vi "Run.vi"(8 "error in (no error)":errorcluster, 11 "Channel in":refnum<class "SPARC4_Channel.lvclass">) -> (0 "error out":errorcluster, 3 "Channel out":refnum<class "SPARC4_Channel.lvclass">)   [LabVIEW 2018, in "SPARC4_Channel.lvclass"]
doc: "Run the channel"
uses:
  SPARC4_Channel.lvclass
  C:/Users/Denis/Desktop/S4ACS/S4ACS/Channel/Channel.lvclass
  Channel/Channel.lvclass/Channel.ctl
  SPARC4_Channel.lvclass/SPARC4_Channel.ctl
  Sim_Ixon_Ultra/Sim_Ixon_Ultra.lvclass
  C:/Users/Denis/Desktop/S4ACS/S4ACS/Sim_CCD/Sim_CCD.lvclass
  State Machine/State Machine.lvclass
  Sim_CCD/Sim_CCD.lvclass
  RxTx/RxTx.lvclass
  Server/Server.lvclass
  Channel/Channel.lvclass
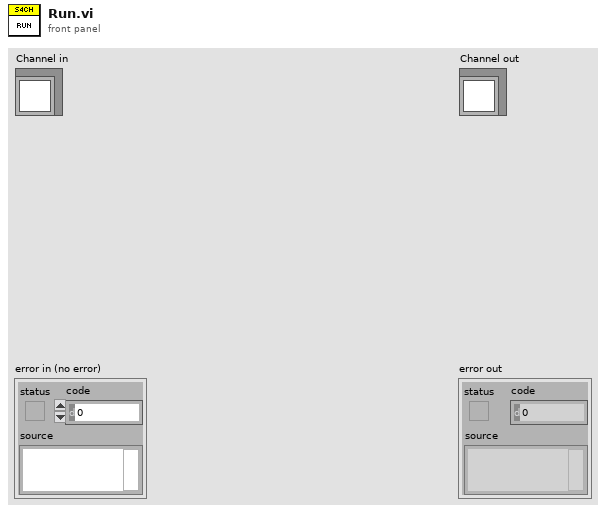
[diagram p1: front panel]
types:
  T1 = cluster{"State Machine.lvclass":refnum<class "State Machine.lvclass">, "RxTx.lvclass":refnum<class "RxTx.lvclass">, "Save_Header_RxTx.lvclass":refnum<class "RxTx.lvclass">, "Status SM.lvclass":refnum<class "State Machine.lvclass">, "Status RxTx.lvclass":refnum<class "RxTx.lvclass">, "servers array":refnum<class "Server.lvclass">[], "Events log file.lvclass":refnum<class "Log File.lvclass">, "Errors log file.lvclass":refnum<class "Log File.lvclass">, "Keywords log file.lvclass":refnum<class "Log File.lvclass">, "Sim_CCD.lvclass":refnum<class "Sim_CCD.lvclass">}
  T2 = cluster{"field 1":string, "field 2":string, "field 3":string}
  T3 = cluster{"PREAMP":u16, "READOUT_RATE":u16, "VERTICAL_SHIFT_SPEED":u16, "READ_MODE":u16, "VERTICAL_CLOCK_VOLTAGE":u16, "ACQUISITION_MODE":u16, "AD_CHANNEL":u16, "SHUTTER_TTL":u16, "SHUTTER_OPENING_TIME":u16, "SHUTTER_CLOSING_TIME":u16, "SHUTTER_MODE":u16, "TRIGGER_MODE":u16, "VBIN":u16, "INITIAL_LINE":u16, "INITIAL_COLUMN":u16, "FINAL_LINE":u16, "FINAL_COLUMN":u16, "HBIN":u16, "TEMP":i32, "COOLER_POWER_STATUS":u16}
  T4 = cluster{"EM_MODE":u16, "EM_GAIN":u16, "FRAME_TRANSFER":bool}
  T5 = typedef "LVDateTimeRec.ctl" = cluster{"fractional second":dbl, "second":i32, "minute":i32, "hour":i32, "day of month":i32, "month":i32, "year":i32, "day of week":i32, "day of year":i32, "DST":i32}
  T6 = cluster{"Time Acq Started":u32, "Image delay":u64, "Last update - CCD config":timestamp, "SYSTEMTIME":T5, "Readout time":dbl, "Time acq finished":u32, "effective exptime":dbl}
  T7 = cluster{"FRAMES_DONE":u16, "CCD_STATUS":string, "CURRENT_TEMPERATURE":i16, "TEMPERATURE_STATUS":string, "FRAME_EXPOSURE_TIME":sgl, "SERIAL_NUMBER":u16, "ACQUIRING":bool, "POWER":bool}
  T8 = cluster{"Stop Acquisition":bool, "Abort Acquisition":bool, "Pause acquisition":bool, "wait expose command":bool, "video mode":bool, "stop app":bool}
  T9 = cluster{"CYCLES_DONE":u16, "LAST_IMAGE_NAME":string, "USED_DISK_SPACE":u16, "IMAGE_INDEX":u32, "acquisition error":bool}
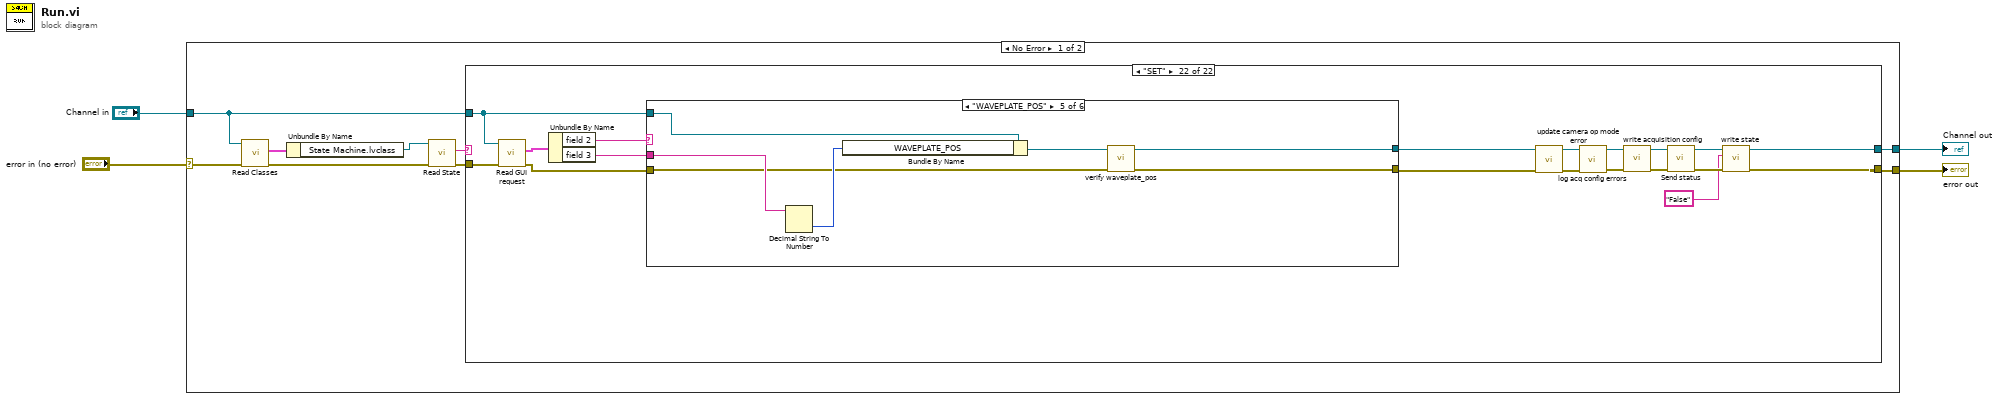
[diagram p0: block diagram]
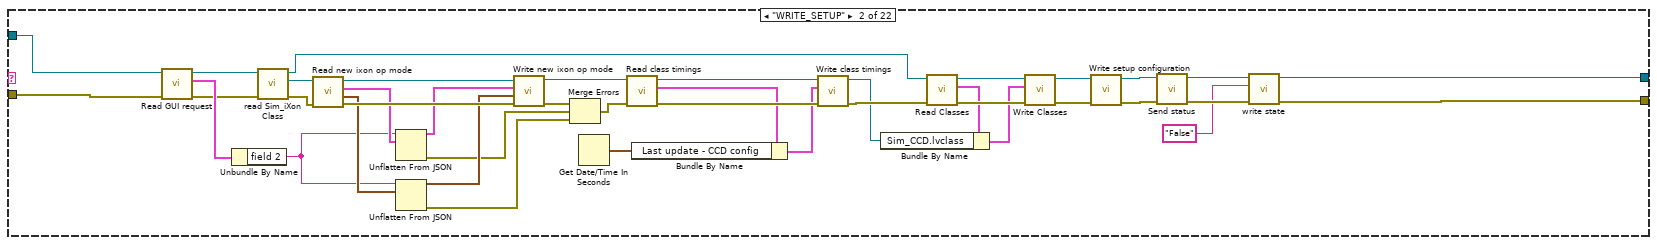
[diagram p3: hidden frame]
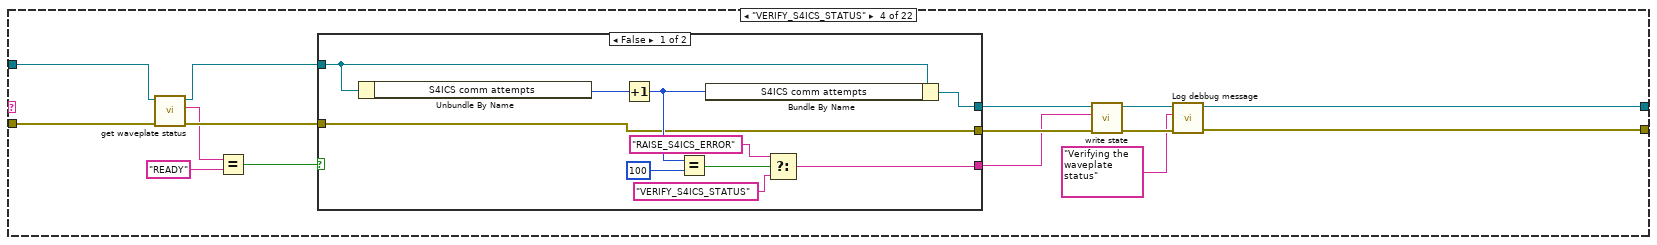
[diagram p5: hidden frame]
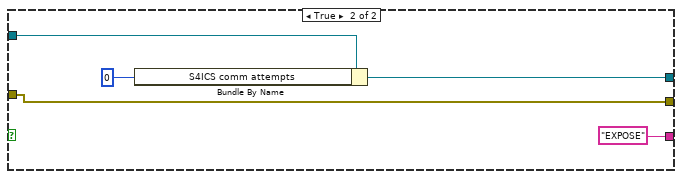
[diagram p6: hidden frame]
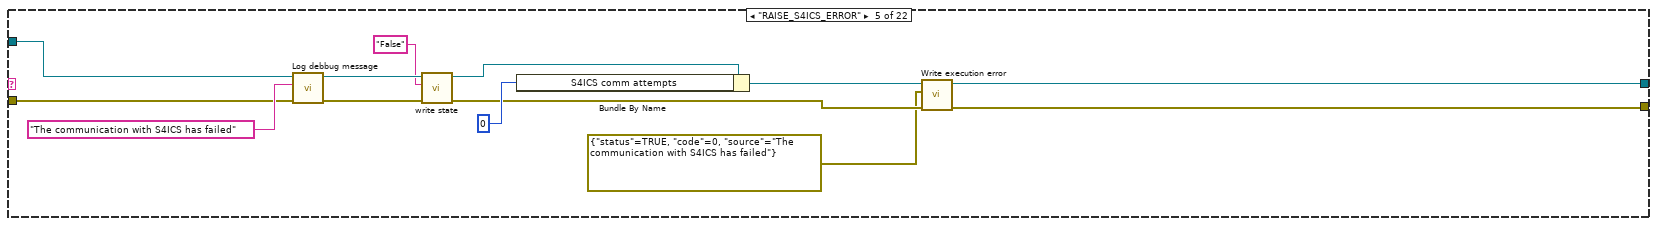
[diagram p7: hidden frame]
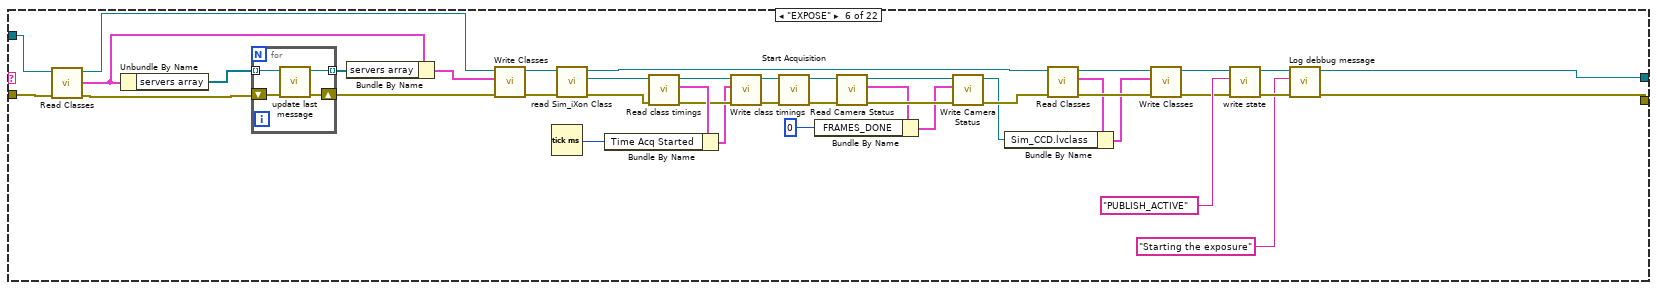
[diagram p8: hidden frame]
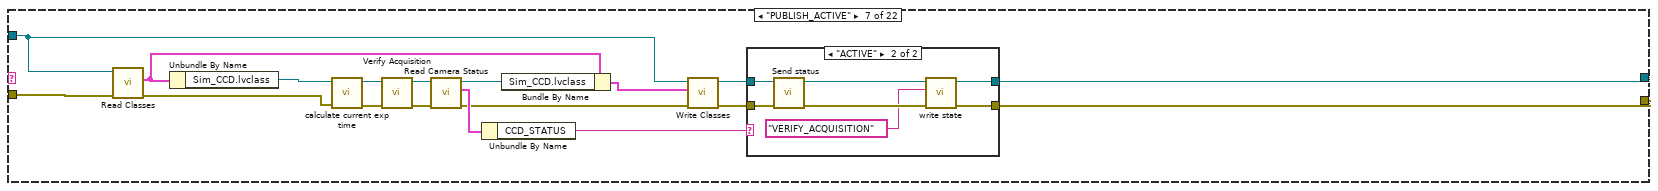
[diagram p9: hidden frame]
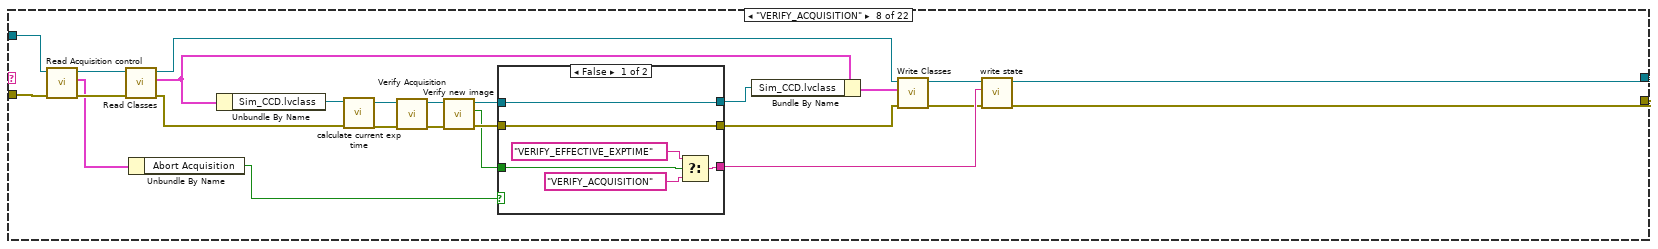
[diagram p11: hidden frame]
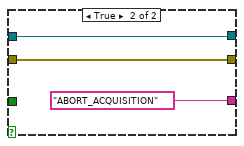
[diagram p12: hidden frame]
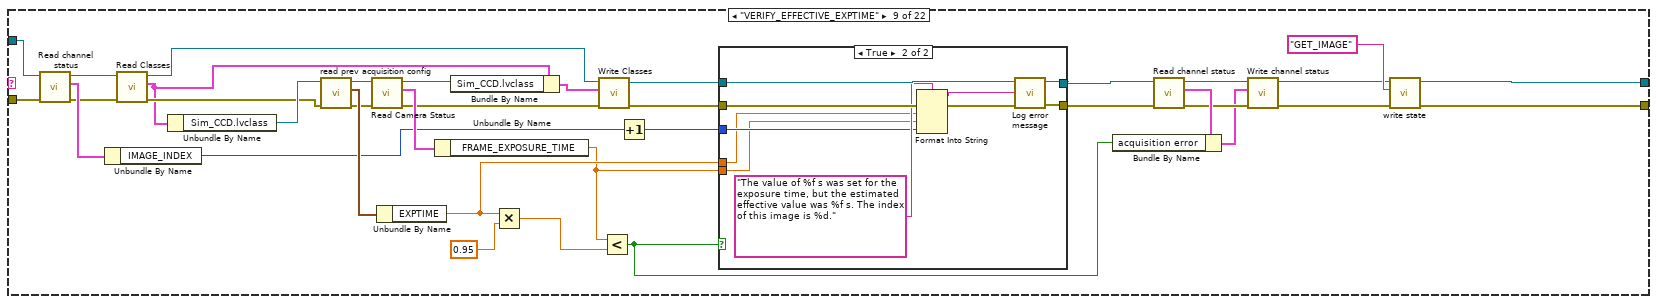
[diagram p13: hidden frame]
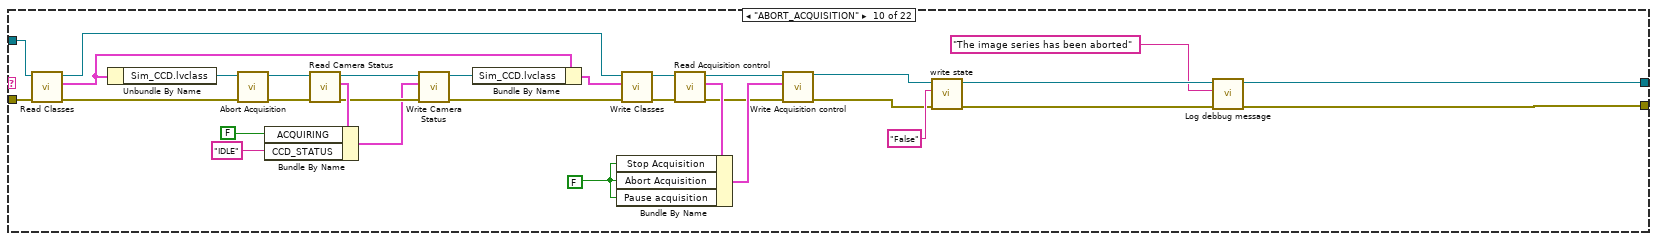
[diagram p15: hidden frame]
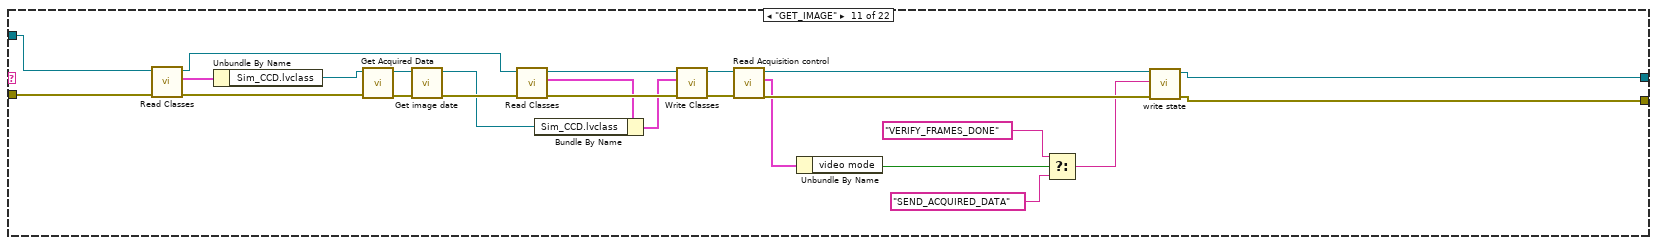
[diagram p16: hidden frame]
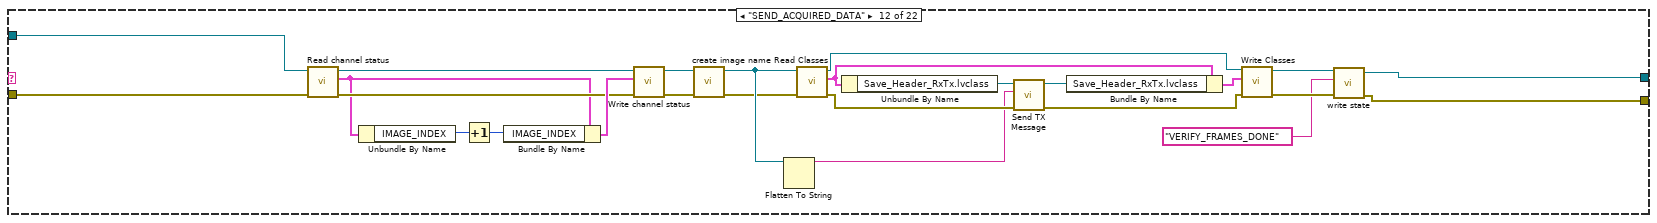
[diagram p17: hidden frame]
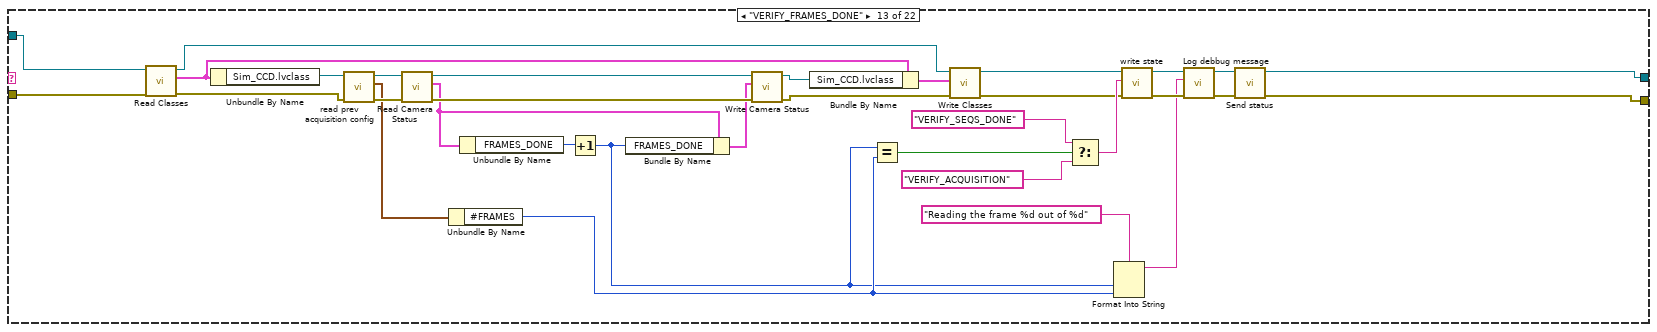
[diagram p18: hidden frame]
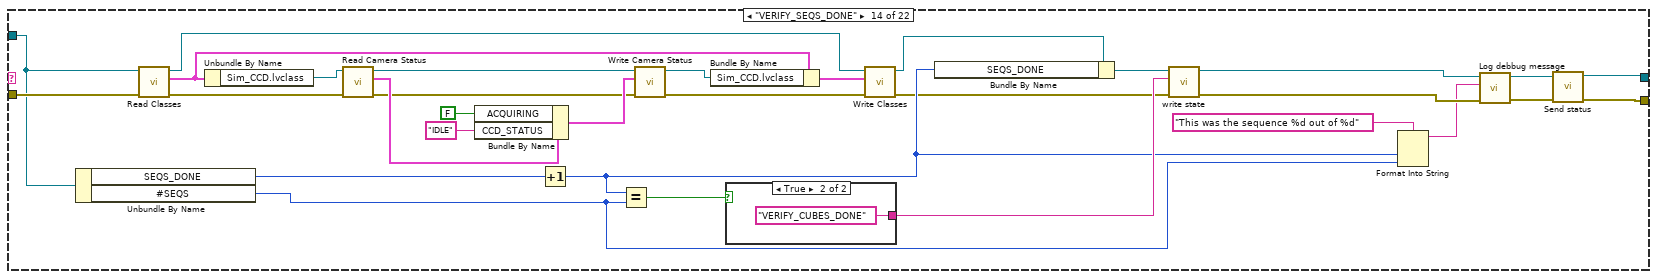
[diagram p19: hidden frame]
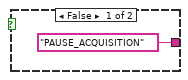
[diagram p20: hidden frame]
diagram:
  n1 = case shown="No Error" "error in (no error)" {
    selector: "error in (no error)" -> [w7 w611]
    tunnel: [w13 w611] -> w3
    tunnel: [w12 w610] -> w1
    tunnel: "Channel in" -> [w8 w610]
    frame No Error {
      n2 = call-dynamic "Read Classes.vi"("error in (no error)"=w7, "Channel in"=w8) -> ("error out"=w6:errorcluster, "Classes"=w9:T1)  [unwired: 7 in, 1 out]
      n3 = Unbundle By Name(w9) -> ("State Machine.lvclass"=w5:refnum<class "State Machine.lvclass">)
      n4 = call-dynamic "Read State.vi"("error in (no error)"=w6, "State Machine in"=w5) -> ("error out"=w11:errorcluster, "State"=w10:string)  [unwired: 7 in, 1 out]
      n5 = case shown="\"SET\"" w10 {
        tunnel: w11 -> [w14 w32 w56 w60 w98 w122 w156 w179 w220 w273 w307 w316 w360 w385 w410 w436 w440 w467 w492 w511 w517 w524]
        tunnel: [w14 w19 w56 w66 w89 w132 w163 w195 w242 w276 w298 w336 w359 w372 w422 w432 w446 w470 w498 w513 w517 w534] -> w13
        tunnel: [w15 w20 w57 w67 w90 w133 w164 w196 w243 w277 w297 w337 w358 w373 w421 w433 w445 w471 w497 w512 w518 w535] -> w12
        tunnel: w8 -> [w15 w34 w57 w62 w99 w121 w151 w177 w214 w272 w308 w317 w361 w381 w408 w437 w441 w468 w493 w510 w518 w523]
        frame "False", Default {
        }
        frame "WRITE_SETUP" {
          n6 = call "Read GUI request.vi"("error in (no error)"=w32, "Channel in"=w34) -> ("error out"=w33:errorcluster, "GUI request"=w39:T2, "Channel out"=w35:refnum<class "SPARC4_Channel.lvclass">)  [unwired: 7 in]
          n7 = Unbundle By Name(w39) -> ("field 2"=w38:string)
          n8 = call "read Sim_iXon Class.vi"("error in (no error)"=w33, "SPARC4_Channel in"=w35) -> ("error out"=w36:errorcluster, "Sim_Ixon_Ultra.lvclass"=w37:refnum<class "Sim_Ixon_Ultra.lvclass">, "SPARC4_Channel out"=w25:refnum<class "SPARC4_Channel.lvclass">)  [unwired: 7 in]
          n9 = call-dynamic "Read new ixon op mode.vi"("error in (no error)"=w36, "Sim_Ixon_Ultra in"=w37) -> ("error out"=w54:errorcluster, "new operation mode"=w53:T3, "new ixon op mode"=w45:T4, "Sim_Ixon_Ultra out"=w55:refnum<class "Sim_Ixon_Ultra.lvclass">)  [unwired: 6 in]
          n10 = Unflatten From JSON(JSON string=w38, type and defaults=w45) -> (value=w44:T4, error out=w41:errorcluster)  [unwired: 5 in]
          n11 = Unflatten From JSON(JSON string=w38, type and defaults=w53) -> (value=w52:T3, error out=w40:errorcluster)  [unwired: 5 in]
          n12 = call-dynamic "Write new ixon op mode.vi"("error in (no error)"=w54, "new operation mode"=w52, "new ixon op mode"=w44, "Sim_Ixon_Ultra in"=w55) -> ("error out"=w43:errorcluster, "Sim_Ixon_Ultra out"=w51:refnum<class "Sim_Ixon_Ultra.lvclass">)  [unwired: 6 in]
          n13 = Merge Errors(w43, w41, w40) -> (w42:errorcluster)
          n14 = Get Date/Time In Seconds() -> (seconds since 1Jan1904=w46:timestamp)
          n15 = call "Read class timings.vi"("error in (no error)"=w42, "Simulated Camera in"=w51) -> ("error out"=w49:errorcluster, "class timings"=w48:T6, "Simulated Camera out"=w50:refnum<class "Sim_Ixon_Ultra.lvclass">)  [unwired: 7 in]
          n16 = Bundle By Name(cluster=w48, "Last update - CCD config"=w46) -> (w47:T6)
          n17 = call "Write class timings.vi"("error in (no error)"=w49, "class timings"=w47, "Simulated Camera in"=w50) -> ("error out"=w29:errorcluster, "Simulated Camera out"=w27:refnum<class "Sim_Ixon_Ultra.lvclass">)  [unwired: 7 in]
          n18 = call-dynamic "Read Classes.vi"("error in (no error)"=w29, "Channel in"=w25) -> ("error out"=w30:errorcluster, "Classes"=w28:T1, "Channel out"=w31:refnum<class "SPARC4_Channel.lvclass">)  [unwired: 7 in]
          n19 = Bundle By Name(cluster=w28, "Sim_CCD.lvclass"=w27) -> (w26:T1)
          n20 = call-dynamic "Write Classes.vi"("error in (no error)"=w30, "Classes"=w26, "Channel in"=w31) -> ("error out"=w21:errorcluster, "Channel out"=w23:refnum<class "SPARC4_Channel.lvclass">)  [unwired: 7 in]
          n21 = call "Write setup configuration.vi"("error in (no error)"=w21, "Channel in"=w23) -> ("error out"=w22:errorcluster, "Channel out"=w24:refnum<class "SPARC4_Channel.lvclass">)  [unwired: 8 in]
          n22 = call-dynamic "Send status.vi"("error in (no error)"=w22, "Channel in"=w24) -> ("error out"=w17:errorcluster, "Channel out"=w18:refnum<class "SPARC4_Channel.lvclass">)  [unwired: 8 in]
          n23 = call "write state.vi"("error in (no error)"=w17, "state"="False", "Channel in"=w18) -> ("error out"=w19:errorcluster, "Channel out"=w20:refnum<class "SPARC4_Channel.lvclass">)  [unwired: 7 in]
        }
        frame "---------------------------------" {
        }
        frame "VERIFY_S4ICS_STATUS" {
          n24 = call "get waveplate status.vi"("error in (no error)"=w60, "Channel in"=w62) -> ("error out"=w59:errorcluster, "wp condition"=w58:string, "Channel out"=w61:refnum<class "SPARC4_Channel.lvclass">)  [unwired: 7 in]
          n25 = Equal?(x=w58, y="READY") -> (x = y?=w71:bool)
          n26 = case shown="False" w71 {
            tunnel: w61 -> [w82 w87]
            tunnel: w59 -> [w75 w86]
            tunnel: [w74 w85] -> w70
            tunnel: [w75 w86] -> w69
            tunnel: [w73 "EXPOSE" ("y")] -> w68
            frame False {
              n27 = Unbundle By Name(w82) -> ("S4ICS comm attempts"=w81:u8)
              n28 = Increment(x=w81) -> (x+1=w80:u8)
              n29 = Equal?(x=w80, y=100) -> (x = y?=w78:bool)
              n30 = Bundle By Name(cluster=w82, "S4ICS comm attempts"=w80) -> (w74:refnum<class "SPARC4_Channel.lvclass">)
              n31 = Select(t="RAISE_S4ICS_ERROR" ("y"), s=w78, f="VERIFY_S4ICS_STATUS" ("y")) -> (s? t:f=w73:string)
            }
            frame True {
              n32 = Bundle By Name(cluster=w87, "S4ICS comm attempts"=u8 0) -> (w85:refnum<class "SPARC4_Channel.lvclass">)
            }
          }
          n33 = call "write state.vi"("error in (no error)"=w69, "state"=w68, "Channel in"=w70) -> ("error out"=w65:errorcluster, "Channel out"=w64:refnum<class "SPARC4_Channel.lvclass">)  [unwired: 7 in]
          n34 = call "Log debbug message.vi"("error in (no error)"=w65, "String"="Verifying the waveplate status" ("y"), "Channel in"=w64) -> ("error out"=w66:errorcluster, "Channel out"=w67:refnum<class "SPARC4_Channel.lvclass">)  [unwired: 7 in]
        }
        frame "RAISE_S4ICS_ERROR" {
          n35 = call "Log debbug message.vi"("error in (no error)"=w98, "String"="The communication with S4ICS has failed", "Channel in"=w99) -> ("error out"=w95:errorcluster, "Channel out"=w96:refnum<class "SPARC4_Channel.lvclass">)  [unwired: 7 in]
          n36 = call "write state.vi"("error in (no error)"=w95, "state"="False", "Channel in"=w96) -> ("error out"=w91:errorcluster, "Channel out"=w94:refnum<class "SPARC4_Channel.lvclass">)  [unwired: 7 in]
          n37 = Bundle By Name(cluster=w94, "S4ICS comm attempts"=u8 0) -> (w92:refnum<class "SPARC4_Channel.lvclass">)
          n38 = call-dynamic "Write execution error.vi"("error in (no error)"=w91, "execution error"=errorcluster {"status"=TRUE, "code"=0, "source"="The communication with S4ICS has failed"} ("error constant"), "Channel in"=w92) -> ("error out"=w89:errorcluster, "Channel out"=w90:refnum<class "SPARC4_Channel.lvclass">)  [unwired: 7 in]
        }
        frame "EXPOSE" {
          n39 = call-dynamic "Read Classes.vi"("error in (no error)"=w122, "Channel in"=w121) -> ("error out"=w118:errorcluster, "Classes"=w115:T1, "Channel out"=w119:refnum<class "SPARC4_Channel.lvclass">)  [unwired: 7 in]
          n40 = Unbundle By Name(w115) -> ("servers array"=w120:refnum<class "Server.lvclass">[])
          n41 = for {
            tunnel: w120 -> [w143] mode=indexing
            shift-right: [w146] -> w117
            shift-left: w118 -> [w144]
            tunnel: [w145] -> w114 mode=indexing
            n42 = call "update last message.vi"("error in (no error)"=w144, "Server in"=w143) -> ("error out"=w146:errorcluster, "Server out"=w145:refnum<class "Server.lvclass">)  [unwired: 8 in]
          }
          n43 = Bundle By Name(cluster=w115, "servers array"=w114) -> (w116:T1)
          n44 = call-dynamic "Write Classes.vi"("error in (no error)"=w117, "Classes"=w116, "Channel in"=w119) -> ("error out"=w111:errorcluster, "Channel out"=w112:refnum<class "SPARC4_Channel.lvclass">)  [unwired: 7 in]
          n45 = Tick Count (ms)() -> (millisecond timer value=w123:u32)
          n46 = call "read Sim_iXon Class.vi"("error in (no error)"=w111, "SPARC4_Channel in"=w112) -> ("error out"=w110:errorcluster, "Sim_Ixon_Ultra.lvclass"=w113:refnum<class "Sim_Ixon_Ultra.lvclass">, "SPARC4_Channel out"=w104:refnum<class "SPARC4_Channel.lvclass">)  [unwired: 7 in]
          n47 = call "Read class timings.vi"("error in (no error)"=w110, "Simulated Camera in"=w113) -> ("error out"=w126:errorcluster, "class timings"=w127:T6, "Simulated Camera out"=w125:refnum<class "Sim_Ixon_Ultra.lvclass">)  [unwired: 7 in]
          n48 = Bundle By Name(cluster=w127, "Time Acq Started"=w123) -> (w124:T6)
          n49 = call "Write class timings.vi"("error in (no error)"=w126, "class timings"=w124, "Simulated Camera in"=w125) -> ("error out"=w129:errorcluster, "Simulated Camera out"=w128:refnum<class "Sim_Ixon_Ultra.lvclass">)  [unwired: 7 in]
          n50 = call-dynamic "Start Acquisition.vi"("error in (no error)"=w129, "CCDCamera in"=w128) -> ("error out"=w135:errorcluster, "CCDCamera out"=w136:refnum<class "Sim_Ixon_Ultra.lvclass">)  [unwired: 8 in]
          n51 = call "Read Camera Status.vi"("error in (no error)"=w135, "CCDCamera in"=w136) -> ("error out"=w142:errorcluster, "camera status"=w140:T7, "CCDCamera out"=w141:refnum<class "Sim_Ixon_Ultra.lvclass">)  [unwired: 7 in]
          n52 = Bundle By Name(cluster=w140, "FRAMES_DONE"=u16 0) -> (w139:T7)
          n53 = call "Write Camera Status.vi"("error in (no error)"=w142, "camera status"=w139, "CCDCamera in"=w141) -> ("error out"=w109:errorcluster, "CCDCamera out"=w101:refnum<class "Sim_Ixon_Ultra.lvclass">)  [unwired: 7 in]
          n54 = call-dynamic "Read Classes.vi"("error in (no error)"=w109, "Channel in"=w104) -> ("error out"=w106:errorcluster, "Classes"=w103:T1, "Channel out"=w105:refnum<class "SPARC4_Channel.lvclass">)  [unwired: 7 in]
          n55 = Bundle By Name(cluster=w103, "Sim_CCD.lvclass"=w101) -> (w102:T1)
          n56 = call-dynamic "Write Classes.vi"("error in (no error)"=w106, "Classes"=w102, "Channel in"=w105) -> ("error out"=w108:errorcluster, "Channel out"=w107:refnum<class "SPARC4_Channel.lvclass">)  [unwired: 7 in]
          n57 = call "write state.vi"("error in (no error)"=w108, "state"="PUBLISH_ACTIVE", "Channel in"=w107) -> ("error out"=w131:errorcluster, "Channel out"=w134:refnum<class "SPARC4_Channel.lvclass">)  [unwired: 7 in]
          n58 = call "Log debbug message.vi"("error in (no error)"=w131, "String"="Starting the exposure", "Channel in"=w134) -> ("error out"=w132:errorcluster, "Channel out"=w133:refnum<class "SPARC4_Channel.lvclass">)  [unwired: 7 in]
        }
        frame "PUBLISH_ACTIVE" {
          n59 = call-dynamic "Read Classes.vi"("error in (no error)"=w156, "Channel in"=w151) -> ("error out"=w154:errorcluster, "Classes"=w149:T1)  [unwired: 7 in, 1 out]
          n60 = Unbundle By Name(w149) -> ("Sim_CCD.lvclass"=w155:refnum<class "Sim_CCD.lvclass">)
          n61 = call-dynamic "calculate current exp time.vi"("error in (no error)"=w154, "CCDCamera in"=w155) -> ("error out"=w157:errorcluster, "CCDCamera out"=w158:refnum<class "Sim_CCD.lvclass">)  [unwired: 8 in]
          n62 = call-dynamic "Verify Acquisition.vi"("error in (no error)"=w157, "CCDCamera in"=w158) -> ("error out"=w159:errorcluster, "CCDCamera out"=w160:refnum<class "Sim_CCD.lvclass">)  [unwired: 8 in]
          n63 = call "Read Camera Status.vi"("error in (no error)"=w159, "CCDCamera in"=w160) -> ("error out"=w150:errorcluster, "camera status"=w162:T7, "CCDCamera out"=w148:refnum<class "Sim_CCD.lvclass">)  [unwired: 7 in]
          n64 = Unbundle By Name(w162) -> ("CCD_STATUS"=w161:string)
          n65 = Bundle By Name(cluster=w149, "Sim_CCD.lvclass"=w148) -> (w147:T1)
          n66 = call-dynamic "Write Classes.vi"("error in (no error)"=w150, "Classes"=w147, "Channel in"=w151) -> ("error out"=w152:errorcluster, "Channel out"=w153:refnum<class "SPARC4_Channel.lvclass">)  [unwired: 7 in]
          n67 = case shown="\"ACTIVE\"" w161 {
            tunnel: w153 -> [w166 w169]
            tunnel: [w166 w173] -> w164
            tunnel: [w165 w172] -> w163
            tunnel: w152 -> [w165 w168]
            frame "False", Default {
            }
            frame "ACTIVE" {
              n68 = call-dynamic "Send status.vi"("error in (no error)"=w168, "Channel in"=w169) -> ("error out"=w171:errorcluster, "Channel out"=w170:refnum<class "SPARC4_Channel.lvclass">)  [unwired: 8 in]
              n69 = call "write state.vi"("error in (no error)"=w171, "state"="VERIFY_ACQUISITION", "Channel in"=w170) -> ("error out"=w172:errorcluster, "Channel out"=w173:refnum<class "SPARC4_Channel.lvclass">)  [unwired: 7 in]
            }
          }
        }
        frame "VERIFY_ACQUISITION" {
          n70 = call "Read Acquisition control.vi"("error in (no error)"=w179, "Channel in"=w177) -> ("error out"=w178:errorcluster, "Acquisition control"=w175:T8, "Channel out"=w176:refnum<class "SPARC4_Channel.lvclass">)  [unwired: 7 in]
          n71 = call-dynamic "Read Classes.vi"("error in (no error)"=w178, "Channel in"=w176) -> ("error out"=w185:errorcluster, "Classes"=w182:T1, "Channel out"=w184:refnum<class "SPARC4_Channel.lvclass">)  [unwired: 7 in]
          n72 = Unbundle By Name(w175) -> ("Abort Acquisition"=w174:bool)
          n73 = Unbundle By Name(w182) -> ("Sim_CCD.lvclass"=w183:refnum<class "Sim_CCD.lvclass">)
          n74 = call-dynamic "calculate current exp time.vi"("error in (no error)"=w185, "CCDCamera in"=w183) -> ("error out"=w191:errorcluster, "CCDCamera out"=w192:refnum<class "Sim_CCD.lvclass">)  [unwired: 8 in]
          n75 = call-dynamic "Verify Acquisition.vi"("error in (no error)"=w191, "CCDCamera in"=w192) -> ("error out"=w198:errorcluster, "CCDCamera out"=w197:refnum<class "Sim_CCD.lvclass">)  [unwired: 8 in]
          n76 = call-dynamic "Verify new image.vi"("error in (no error)"=w198, "CCDCamera in"=w197) -> ("error out"=w193:errorcluster, "New Images ?"=w189:bool, "CCDCamera out"=w194:refnum<class "Sim_CCD.lvclass">)  [unwired: 7 in]
          n77 = case shown="False" w174 {
            tunnel: w194 -> [w204 w207]
            tunnel: w193 -> [w203 w206]
            tunnel: [w204 w207] -> w180
            tunnel: [w203 w206] -> w186
            tunnel: [w200 "ABORT_ACQUISITION"] -> w190
            tunnel: w189 -> [w199 _]
            frame False {
              n78 = Select(t="VERIFY_EFFECTIVE_EXPTIME", s=w199, f="VERIFY_ACQUISITION") -> (s? t:f=w200:string)
            }
            frame True {
            }
          }
          n79 = Bundle By Name(cluster=w182, "Sim_CCD.lvclass"=w180) -> (w181:T1)
          n80 = call-dynamic "Write Classes.vi"("error in (no error)"=w186, "Classes"=w181, "Channel in"=w184) -> ("error out"=w188:errorcluster, "Channel out"=w187:refnum<class "SPARC4_Channel.lvclass">)  [unwired: 7 in]
          n81 = call "write state.vi"("error in (no error)"=w188, "state"=w190, "Channel in"=w187) -> ("error out"=w195:errorcluster, "Channel out"=w196:refnum<class "SPARC4_Channel.lvclass">)  [unwired: 7 in]
        }
        frame "VERIFY_EFFECTIVE_EXPTIME" {
          n82 = call-dynamic "Read channel status.vi"("error in (no error)"=w220, "Channel in"=w214) -> ("error out"=w219:errorcluster, "channel status"=w222:T9, "Channel out"=w218:refnum<class "SPARC4_Channel.lvclass">)  [unwired: 7 in]
          n83 = Unbundle By Name(w222) -> ("IMAGE_INDEX"=w221:u32)
          n84 = call-dynamic "Read Classes.vi"("error in (no error)"=w219, "Channel in"=w218) -> ("error out"=w216:errorcluster, "Classes"=w210:T1, "Channel out"=w213:refnum<class "SPARC4_Channel.lvclass">)  [unwired: 7 in]
          n85 = Unbundle By Name(w210) -> ("Sim_CCD.lvclass"=w217:refnum<class "Sim_CCD.lvclass">)
          n86 = call "read prev acquisition config.vi"("error in (no error)"=w216, "Simulated_CCD_Camera in"=w217) -> ("error out"=w236:errorcluster, "Prev SET parameters"=w238:cluster{"EXPTIME":dbl, "#FRAMES":u32}, "Simulated_CCD_Camera out"=w237:refnum<class "Sim_CCD.lvclass">)  [unwired: 7 in]
          n87 = call "Read Camera Status.vi"("error in (no error)"=w236, "CCDCamera in"=w237) -> ("error out"=w211:errorcluster, "camera status"=w235:T7, "CCDCamera out"=w208:refnum<class "Sim_CCD.lvclass">)  [unwired: 7 in]
          n88 = Unbundle By Name(w238) -> ("EXPTIME"=w233:dbl)
          n89 = Unbundle By Name(w235) -> ("FRAME_EXPOSURE_TIME"=w232:sgl)
          n90 = Bundle By Name(cluster=w210, "Sim_CCD.lvclass"=w208) -> (w209:T1)
          n91 = Multiply(x=w233, y=0.95) -> (x*y=w239:dbl)
          n92 = call-dynamic "Write Classes.vi"("error in (no error)"=w211, "Classes"=w209, "Channel in"=w213) -> ("error out"=w215:errorcluster, "Channel out"=w212:refnum<class "SPARC4_Channel.lvclass">)  [unwired: 7 in]
          n93 = Less?(x=w232, y=w239) -> (x < y?=w230:bool)
          n94 = Increment(x=w221) -> (x+1=w234:u32)
          n95 = case shown="True" w230 {
            tunnel: w212 -> [w245 w255]
            tunnel: [w245 w254] -> w229
            tunnel: [w244 w253] -> w228
            tunnel: w215 -> [w244 w252]
            tunnel: w234 -> [_ w248]
            tunnel: w233 -> [_ w247]
            tunnel: w232 -> [_ w246]
            frame False {
            }
            frame True {
              n96 = Format Into String(format string="The value of %f s was set for the exposure time, but the estimated effective value was %f s. The index of this image is %d.", error in=w252, w247, w246, w248) -> (resulting string=w249:string, error out=w251:errorcluster)  [unwired: 1 in]
              n97 = call "Log error message.vi"("error in (no error)"=w251, "String"=w249, "Channel in"=w255) -> ("error out"=w253:errorcluster, "Channel out"=w254:refnum<class "SPARC4_Channel.lvclass">)  [unwired: 7 in]
            }
          }
          n98 = call-dynamic "Read channel status.vi"("error in (no error)"=w228, "Channel in"=w229) -> ("error out"=w224:errorcluster, "channel status"=w231:T9, "Channel out"=w225:refnum<class "SPARC4_Channel.lvclass">)  [unwired: 7 in]
          n99 = Bundle By Name(cluster=w231, "acquisition error"=w230) -> (w223:T9)
          n100 = call-dynamic "Write channel status.vi"("error in (no error)"=w224, "channel status"=w223, "Channel in"=w225) -> ("error out"=w227:errorcluster, "Channel out"=w226:refnum<class "SPARC4_Channel.lvclass">)  [unwired: 7 in]
          n101 = call "write state.vi"("error in (no error)"=w227, "state"="GET_IMAGE", "Channel in"=w226) -> ("error out"=w242:errorcluster, "Channel out"=w243:refnum<class "SPARC4_Channel.lvclass">)  [unwired: 7 in]
        }
        frame "ABORT_ACQUISITION" {
          w256 = FALSE ("Acquiring")
          n102 = call-dynamic "Read Classes.vi"("error in (no error)"=w273, "Channel in"=w272) -> ("error out"=w270:errorcluster, "Classes"=w266:T1, "Channel out"=w265:refnum<class "SPARC4_Channel.lvclass">)  [unwired: 7 in]
          n103 = Unbundle By Name(w266) -> ("Sim_CCD.lvclass"=w271:refnum<class "Sim_CCD.lvclass">)
          n104 = call-dynamic "Abort Acquisition.vi"("error in (no error)"=w270, "CCDCamera in"=w271) -> ("error out"=w284:errorcluster, "CCDCamera out"=w285:refnum<class "Sim_CCD.lvclass">)  [unwired: 8 in]
          n105 = call "Read Camera Status.vi"("error in (no error)"=w284, "CCDCamera in"=w285) -> ("error out"=w282:errorcluster, "camera status"=w287:T7, "CCDCamera out"=w283:refnum<class "Sim_CCD.lvclass">)  [unwired: 7 in]
          n106 = Bundle By Name(cluster=w287, "ACQUIRING"=FALSE ("Acquiring"), "CCD_STATUS"="IDLE" ("STATUS")) -> (w281:T7)
          n107 = call "Write Camera Status.vi"("error in (no error)"=w282, "camera status"=w281, "CCDCamera in"=w283) -> ("error out"=w268:errorcluster, "CCDCamera out"=w269:refnum<class "Sim_CCD.lvclass">)  [unwired: 7 in]
          n108 = Bundle By Name(cluster=w266, "Sim_CCD.lvclass"=w269) -> (w267:T1)
          n109 = call-dynamic "Write Classes.vi"("error in (no error)"=w268, "Classes"=w267, "Channel in"=w265) -> ("error out"=w263:errorcluster, "Channel out"=w264:refnum<class "SPARC4_Channel.lvclass">)  [unwired: 7 in]
          n110 = call "Read Acquisition control.vi"("error in (no error)"=w263, "Channel in"=w264) -> ("error out"=w257:errorcluster, "Acquisition control"=w259:T8, "Channel out"=w262:refnum<class "SPARC4_Channel.lvclass">)  [unwired: 7 in]
          n111 = Bundle By Name(cluster=w259, "Stop Acquisition"=w256, "Abort Acquisition"=w256, "Pause acquisition"=w256) -> (w258:T8)
          n112 = call "Write Acquisition control.vi"("error in (no error)"=w257, "Acquisition control"=w258, "Channel in"=w262) -> ("error out"=w260:errorcluster, "Channel out"=w261:refnum<class "SPARC4_Channel.lvclass">)  [unwired: 7 in]
          n113 = call "write state.vi"("error in (no error)"=w260, "state"="False", "Channel in"=w261) -> ("error out"=w275:errorcluster, "Channel out"=w278:refnum<class "SPARC4_Channel.lvclass">)  [unwired: 7 in]
          n114 = call "Log debbug message.vi"("error in (no error)"=w275, "String"="The image series has been aborted", "Channel in"=w278) -> ("error out"=w276:errorcluster, "Channel out"=w277:refnum<class "SPARC4_Channel.lvclass">)  [unwired: 7 in]
        }
        frame "GET_IMAGE" {
          n115 = call-dynamic "Read Classes.vi"("error in (no error)"=w307, "Channel in"=w308) -> ("error out"=w305:errorcluster, "Classes"=w306:T1, "Channel out"=w303:refnum<class "SPARC4_Channel.lvclass">)  [unwired: 7 in]
          n116 = Unbundle By Name(w306) -> ("Sim_CCD.lvclass"=w304:refnum<class "Sim_CCD.lvclass">)
          n117 = call-dynamic "Get Acquired Data.vi"("error in (no error)"=w305, "CCDCamera in"=w304) -> ("error out"=w311:errorcluster, "CCDCamera out"=w312:refnum<class "Sim_CCD.lvclass">)  [unwired: 8 in]
          n118 = call-dynamic "Get image date.vi"("error in (no error)"=w311, "Simulated_CCD_Camera in"=w312) -> ("error out"=w310:errorcluster, "Simulated_CCD_Camera out"=w309:refnum<class "Sim_CCD.lvclass">)  [unwired: 8 in]
          n119 = call-dynamic "Read Classes.vi"("error in (no error)"=w310, "Channel in"=w303) -> ("error out"=w302:errorcluster, "Classes"=w301:T1, "Channel out"=w300:refnum<class "SPARC4_Channel.lvclass">)  [unwired: 7 in]
          n120 = Bundle By Name(cluster=w301, "Sim_CCD.lvclass"=w309) -> (w299:T1)
          n121 = call-dynamic "Write Classes.vi"("error in (no error)"=w302, "Classes"=w299, "Channel in"=w300) -> ("error out"=w295:errorcluster, "Channel out"=w296:refnum<class "SPARC4_Channel.lvclass">)  [unwired: 7 in]
          n122 = call "Read Acquisition control.vi"("error in (no error)"=w295, "Channel in"=w296) -> ("error out"=w293:errorcluster, "Acquisition control"=w292:T8, "Channel out"=w294:refnum<class "SPARC4_Channel.lvclass">)  [unwired: 7 in]
          n123 = Unbundle By Name(w292) -> ("video mode"=w291:bool)
          n124 = Select(t="VERIFY_FRAMES_DONE", s=w291, f="SEND_ACQUIRED_DATA") -> (s? t:f=w288:string)
          n125 = call "write state.vi"("error in (no error)"=w293, "state"=w288, "Channel in"=w294) -> ("error out"=w298:errorcluster, "Channel out"=w297:refnum<class "SPARC4_Channel.lvclass">)  [unwired: 7 in]
        }
        frame "SEND_ACQUIRED_DATA" {
          n126 = call-dynamic "Read channel status.vi"("error in (no error)"=w316, "Channel in"=w317) -> ("error out"=w323:errorcluster, "channel status"=w315:T9, "Channel out"=w322:refnum<class "SPARC4_Channel.lvclass">)  [unwired: 7 in]
          n127 = Unbundle By Name(w315) -> ("IMAGE_INDEX"=w314:u32)
          n128 = Increment(x=w314) -> (x+1=w313:u32)
          n129 = Bundle By Name(cluster=w315, "IMAGE_INDEX"=w313) -> (w324:T9)
          n130 = call-dynamic "Write channel status.vi"("error in (no error)"=w323, "channel status"=w324, "Channel in"=w322) -> ("error out"=w318:errorcluster, "Channel out"=w319:refnum<class "SPARC4_Channel.lvclass">)  [unwired: 7 in]
          n131 = call-dynamic "create image name.vi"("error in (no error)"=w318, "Channel in"=w319) -> ("error out"=w320:errorcluster, "Channel out"=w321:refnum<class "SPARC4_Channel.lvclass">)  [unwired: 8 in]
          n132 = Flatten To String(anything=w321) -> (data string=w326:string)  [unwired: 3 in, 2 out]
          n133 = call-dynamic "Read Classes.vi"("error in (no error)"=w320, "Channel in"=w321) -> ("error out"=w331:errorcluster, "Classes"=w330:T1, "Channel out"=w325:refnum<class "SPARC4_Channel.lvclass">)  [unwired: 7 in]
          n134 = Unbundle By Name(w330) -> ("Save_Header_RxTx.lvclass"=w332:refnum<class "RxTx.lvclass">)
          n135 = call "Send TX Message.vi"("error in (no error)"=w331, "message"=w326, "RxTx in"=w332) -> ("error out"=w327:errorcluster, "RxTx out"=w328:refnum<class "RxTx.lvclass">)  [unwired: 7 in]
          n136 = Bundle By Name(cluster=w330, "Save_Header_RxTx.lvclass"=w328) -> (w329:T1)
          n137 = call-dynamic "Write Classes.vi"("error in (no error)"=w327, "Classes"=w329, "Channel in"=w325) -> ("error out"=w335:errorcluster, "Channel out"=w334:refnum<class "SPARC4_Channel.lvclass">)  [unwired: 7 in]
          n138 = call "write state.vi"("error in (no error)"=w335, "state"="VERIFY_FRAMES_DONE", "Channel in"=w334) -> ("error out"=w336:errorcluster, "Channel out"=w337:refnum<class "SPARC4_Channel.lvclass">)  [unwired: 7 in]
        }
        frame "VERIFY_FRAMES_DONE" {
          n139 = call-dynamic "Read Classes.vi"("error in (no error)"=w360, "Channel in"=w361) -> ("error out"=w342:errorcluster, "Classes"=w363:T1, "Channel out"=w362:refnum<class "SPARC4_Channel.lvclass">)  [unwired: 7 in]
          n140 = Unbundle By Name(w363) -> ("Sim_CCD.lvclass"=w343:refnum<class "Sim_CCD.lvclass">)
          n141 = call "read prev acquisition config.vi"("error in (no error)"=w342, "Simulated_CCD_Camera in"=w343) -> ("error out"=w348:errorcluster, "Prev SET parameters"=w346:cluster{"EXPTIME":dbl, "#FRAMES":u32}, "Simulated_CCD_Camera out"=w347:refnum<class "Sim_CCD.lvclass">)  [unwired: 7 in]
          n142 = call "Read Camera Status.vi"("error in (no error)"=w348, "CCDCamera in"=w347) -> ("error out"=w353:errorcluster, "camera status"=w349:T7, "CCDCamera out"=w352:refnum<class "Sim_CCD.lvclass">)  [unwired: 7 in]
          n143 = Unbundle By Name(w346) -> ("#FRAMES"=w339:u32)
          n144 = Unbundle By Name(w349) -> ("FRAMES_DONE"=w351:u16)
          n145 = Increment(x=w351) -> (x+1=w338:u16)
          n146 = Bundle By Name(cluster=w349, "FRAMES_DONE"=w338) -> (w350:T7)
          n147 = call "Write Camera Status.vi"("error in (no error)"=w353, "camera status"=w350, "CCDCamera in"=w352) -> ("error out"=w340:errorcluster, "CCDCamera out"=w341:refnum<class "Sim_CCD.lvclass">)  [unwired: 7 in]
          n148 = Bundle By Name(cluster=w363, "Sim_CCD.lvclass"=w341) -> (w364:T1)
          n149 = Equal?(x=w338, y=w339) -> (x = y?=w370:bool)
          n150 = call-dynamic "Write Classes.vi"("error in (no error)"=w340, "Classes"=w364, "Channel in"=w362) -> ("error out"=w365:errorcluster, "Channel out"=w366:refnum<class "SPARC4_Channel.lvclass">)  [unwired: 7 in]
          n151 = Select(t="VERIFY_SEQS_DONE", s=w370, f="VERIFY_ACQUISITION") -> (s? t:f=w367:string)
          n152 = Format Into String(format string="Reading the frame %d out of %d", w338, w339) -> (resulting string=w344:string)  [unwired: 2 in, 1 out]
          n153 = call "write state.vi"("error in (no error)"=w365, "state"=w367, "Channel in"=w366) -> ("error out"=w354:errorcluster, "Channel out"=w357:refnum<class "SPARC4_Channel.lvclass">)  [unwired: 7 in]
          n154 = call "Log debbug message.vi"("error in (no error)"=w354, "String"=w344, "Channel in"=w357) -> ("error out"=w355:errorcluster, "Channel out"=w356:refnum<class "SPARC4_Channel.lvclass">)  [unwired: 7 in]
          n155 = call-dynamic "Send status.vi"("error in (no error)"=w355, "Channel in"=w356) -> ("error out"=w359:errorcluster, "Channel out"=w358:refnum<class "SPARC4_Channel.lvclass">)  [unwired: 8 in]
        }
        frame "VERIFY_SEQS_DONE" {
          n156 = Unbundle By Name(w381) -> ("SEQS_DONE"=w388:u16, "#SEQS"=w386:u32)
          n157 = call-dynamic "Read Classes.vi"("error in (no error)"=w385, "Channel in"=w381) -> ("error out"=w384:errorcluster, "Classes"=w377:T1, "Channel out"=w380:refnum<class "SPARC4_Channel.lvclass">)  [unwired: 7 in]
          n158 = Unbundle By Name(w377) -> ("Sim_CCD.lvclass"=w383:refnum<class "Sim_CCD.lvclass">)
          n159 = call "Read Camera Status.vi"("error in (no error)"=w384, "CCDCamera in"=w383) -> ("error out"=w397:errorcluster, "camera status"=w401:T7, "CCDCamera out"=w398:refnum<class "Sim_CCD.lvclass">)  [unwired: 7 in]
          n160 = Bundle By Name(cluster=w401, "ACQUIRING"=FALSE, "CCD_STATUS"="IDLE") -> (w400:T7)
          n161 = Increment(x=w388) -> (x+1=w387:u16)
          n162 = Equal?(x=w387, y=w386) -> (x = y?=w399:bool)
          n163 = call "Write Camera Status.vi"("error in (no error)"=w397, "camera status"=w400, "CCDCamera in"=w398) -> ("error out"=w378:errorcluster, "CCDCamera out"=w375:refnum<class "Sim_CCD.lvclass">)  [unwired: 7 in]
          n164 = Bundle By Name(cluster=w377, "Sim_CCD.lvclass"=w375) -> (w376:T1)
          n165 = case shown="True" w399 {
            tunnel: ["PAUSE_ACQUISITION" "VERIFY_CUBES_DONE"] -> w393
            frame False {
            }
            frame True {
            }
          }
          n166 = call-dynamic "Write Classes.vi"("error in (no error)"=w378, "Classes"=w376, "Channel in"=w380) -> ("error out"=w379:errorcluster, "Channel out"=w382:refnum<class "SPARC4_Channel.lvclass">)  [unwired: 7 in]
          n167 = Bundle By Name(cluster=w382, "SEQS_DONE"=w387) -> (w394:refnum<class "SPARC4_Channel.lvclass">)
          n168 = call "write state.vi"("error in (no error)"=w379, "state"=w393, "Channel in"=w394) -> ("error out"=w391:errorcluster, "Channel out"=w392:refnum<class "SPARC4_Channel.lvclass">)  [unwired: 7 in]
          n169 = Format Into String(format string="This was the sequence %d out of %d", w387, w386) -> (resulting string=w389:string)  [unwired: 2 in, 1 out]
          n170 = call "Log debbug message.vi"("error in (no error)"=w391, "String"=w389, "Channel in"=w392) -> ("error out"=w371:errorcluster, "Channel out"=w374:refnum<class "SPARC4_Channel.lvclass">)  [unwired: 7 in]
          n171 = call-dynamic "Send status.vi"("error in (no error)"=w371, "Channel in"=w374) -> ("error out"=w372:errorcluster, "Channel out"=w373:refnum<class "SPARC4_Channel.lvclass">)  [unwired: 8 in]
        }
        frame "VERIFY_CUBES_DONE" {
          n172 = call-dynamic "Read prev acq config.vi"("error in (no error)"=w410, "Channel in"=w408) -> ("error out"=w409:errorcluster, "prev acq config"=w416:cluster{"suffix":string, "#CYCLES":u32}, "Channel out"=w407:refnum<class "SPARC4_Channel.lvclass">)  [unwired: 7 in]
          n173 = call-dynamic "Read channel status.vi"("error in (no error)"=w409, "Channel in"=w407) -> ("error out"=w406:errorcluster, "channel status"=w413:T9, "Channel out"=w405:refnum<class "SPARC4_Channel.lvclass">)  [unwired: 7 in]
          n174 = Unbundle By Name(w416) -> ("#CYCLES"=w415:u32)
          n175 = Unbundle By Name(w413) -> ("CYCLES_DONE"=w417:u16)
          n176 = Increment(x=w417) -> (x+1=w412:u16)
          n177 = Equal?(x=w412, y=w415) -> (x = y?=w427:bool)
          n178 = case shown="True" w427 {
            tunnel: ["PAUSE_ACQUISITION" "LOG_END_OF_SERIES"] -> w424
            frame False {
            }
            frame True {
            }
          }
          n179 = Bundle By Name(cluster=w413, "CYCLES_DONE"=w412) -> (w411:T9)
          n180 = call-dynamic "Write channel status.vi"("error in (no error)"=w406, "channel status"=w411, "Channel in"=w405) -> ("error out"=w414:errorcluster, "Channel out"=w404:refnum<class "SPARC4_Channel.lvclass">)  [unwired: 7 in]
          n181 = call "write state.vi"("error in (no error)"=w414, "state"=w424, "Channel in"=w404) -> ("error out"=w425:errorcluster, "Channel out"=w426:refnum<class "SPARC4_Channel.lvclass">)  [unwired: 7 in]
          n182 = Format Into String(format string="This was the cycle %d out of %d", w412, w415) -> (resulting string=w419:string)  [unwired: 2 in, 1 out]
          n183 = call-dynamic "Send status.vi"("error in (no error)"=w425, "Channel in"=w426) -> ("error out"=w423:errorcluster, "Channel out"=w420:refnum<class "SPARC4_Channel.lvclass">)  [unwired: 8 in]
          n184 = call "Log debbug message.vi"("error in (no error)"=w423, "String"=w419, "Channel in"=w420) -> ("error out"=w422:errorcluster, "Channel out"=w421:refnum<class "SPARC4_Channel.lvclass">)  [unwired: 7 in]
        }
        frame "LOG_END_OF_SERIES" {
          n185 = call "write state.vi"("error in (no error)"=w436, "state"="False", "Channel in"=w437) -> ("error out"=w434:errorcluster, "Channel out"=w435:refnum<class "SPARC4_Channel.lvclass">)  [unwired: 7 in]
          n186 = call "Log info message.vi"("error in (no error)"=w434, "String"="The acquisition of the image series has been finished", "Channel in"=w435) -> ("error out"=w432:errorcluster, "Channel out"=w433:refnum<class "SPARC4_Channel.lvclass">)  [unwired: 7 in]
        }
        frame "PAUSE_ACQUISITION" {
          n187 = call "Read Acquisition control.vi"("error in (no error)"=w440, "Channel in"=w441) -> ("error out"=w439:errorcluster, "Acquisition control"=w443:T8, "Channel out"=w438:refnum<class "SPARC4_Channel.lvclass">)  [unwired: 7 in]
          n188 = Unbundle By Name(w443) -> ("Pause acquisition"=w442:bool)
          n189 = Select(t="PAUSE_ACQUISITION", s=w442, f="STOP_ACQUISITION") -> (s? t:f=w444:string)
          n190 = call "write state.vi"("error in (no error)"=w439, "state"=w444, "Channel in"=w438) -> ("error out"=w446:errorcluster, "Channel out"=w445:refnum<class "SPARC4_Channel.lvclass">)  [unwired: 7 in]
        }
        frame "STOP_ACQUISITION" {
          n191 = call "Read Acquisition control.vi"("error in (no error)"=w467, "Channel in"=w468) -> ("error out"=w466:errorcluster, "Acquisition control"=w465:T8, "Channel out"=w462:refnum<class "SPARC4_Channel.lvclass">)  [unwired: 7 in]
          n192 = Bundle By Name(cluster=w465, "Stop Acquisition"=FALSE) -> (w464:T8)
          n193 = Unbundle By Name(w465) -> ("Stop Acquisition"=w469:bool)
          n194 = call "Write Acquisition control.vi"("error in (no error)"=w466, "Acquisition control"=w464, "Channel in"=w462) -> ("error out"=w460:errorcluster, "Channel out"=w461:refnum<class "SPARC4_Channel.lvclass">)  [unwired: 7 in]
          n195 = Select(t="False", s=w469, f="WAIT_EXPOSE_COMMAND") -> (s? t:f=w472:string)
          n196 = call "write state.vi"("error in (no error)"=w460, "state"=w472, "Channel in"=w461) -> ("error out"=w459:errorcluster, "Channel out"=w458:refnum<class "SPARC4_Channel.lvclass">)  [unwired: 7 in]
          n197 = call-dynamic "Read Classes.vi"("error in (no error)"=w459, "Channel in"=w458) -> ("error out"=w456:errorcluster, "Classes"=w453:T1, "Channel out"=w452:refnum<class "SPARC4_Channel.lvclass">)  [unwired: 7 in]
          n198 = Not(x=w469) -> (.not. x?=w473:bool)
          n199 = Unbundle By Name(w453) -> ("Sim_CCD.lvclass"=w457:refnum<class "Sim_CCD.lvclass">)
          n200 = Select(t="WAITING_EXPOSE_COMMAND" ("CCD_STATUS"), s=w473, f="IDLE" ("CCD_STATUS")) -> (s? t:f=w476:string)
          n201 = call "Read Camera Status.vi"("error in (no error)"=w456, "CCDCamera in"=w457) -> ("error out"=w478:errorcluster, "camera status"=w480:T7, "CCDCamera out"=w477:refnum<class "Sim_CCD.lvclass">)  [unwired: 7 in]
          n202 = Bundle By Name(cluster=w480, "CCD_STATUS"=w476) -> (w479:T7)
          n203 = call "Write Camera Status.vi"("error in (no error)"=w478, "camera status"=w479, "CCDCamera in"=w477) -> ("error out"=w455:errorcluster, "CCDCamera out"=w451:refnum<class "Sim_CCD.lvclass">)  [unwired: 7 in]
          n204 = Bundle By Name(cluster=w453, "Sim_CCD.lvclass"=w451) -> (w454:T1)
          n205 = call-dynamic "Write Classes.vi"("error in (no error)"=w455, "Classes"=w454, "Channel in"=w452) -> ("error out"=w449:errorcluster, "Channel out"=w450:refnum<class "SPARC4_Channel.lvclass">)  [unwired: 7 in]
          n206 = case shown="True" w469 {
            tunnel: w450 -> [w484 w489]
            tunnel: [w484 w488] -> w471
            tunnel: [w483 w487] -> w470
            tunnel: w449 -> [w483 w486]
            frame False {
            }
            frame True {
              n207 = call "Log debbug message.vi"("error in (no error)"=w486, "String"="The acquisition has been stopped", "Channel in"=w489) -> ("error out"=w487:errorcluster, "Channel out"=w488:refnum<class "SPARC4_Channel.lvclass">)  [unwired: 7 in]
            }
          }
        }
        frame "WAIT_EXPOSE_COMMAND" {
          n208 = call "Read Acquisition control.vi"("error in (no error)"=w492, "Channel in"=w493) -> ("error out"=w490:errorcluster, "Acquisition control"=w495:T8, "Channel out"=w491:refnum<class "SPARC4_Channel.lvclass">)  [unwired: 7 in]
          n209 = Unbundle By Name(w495) -> ("wait expose command"=w494:bool)
          n210 = Select(t="STOP_ACQUISITION", s=w494, f="RESET_#SEQS") -> (s? t:f=w496:string)
          n211 = call "write state.vi"("error in (no error)"=w490, "state"=w496, "Channel in"=w491) -> ("error out"=w498:errorcluster, "Channel out"=w497:refnum<class "SPARC4_Channel.lvclass">)  [unwired: 7 in]
        }
        frame "RESET_#SEQS" {
          n212 = call "choose firs acquisition state.vi"("error in (no error)"=w511, "Channel in"=w510) -> ("error out"=w508:errorcluster, "verify S4ICS status"=w504:bool, "Channel out"=w509:refnum<class "SPARC4_Channel.lvclass">)  [unwired: 7 in]
          n213 = Select(t="VERIFY_S4ICS_STATUS", s=w504, f="EXPOSE") -> (s? t:f=w506:string)
          n214 = call "write state.vi"("error in (no error)"=w508, "state"=w506, "Channel in"=w509) -> ("error out"=w513:errorcluster, "Channel out"=w514:refnum<class "SPARC4_Channel.lvclass">)  [unwired: 7 in]
          n215 = Unbundle By Name(w514) -> ("#SEQS"=w502:u32, "SEQS_DONE"=w501:u16)
          n216 = Equal?(x=w502, y=w501) -> (x = y?=w516:bool)
          n217 = Select(t=0, s=w516, f=w501) -> (s? t:f=w503:i32)
          n218 = Bundle By Name(cluster=w514, "SEQS_DONE"=w503) -> (w512:refnum<class "SPARC4_Channel.lvclass">)
        }
        frame "------------------------------" {
        }
        frame "SET" {
          n219 = call "Read GUI request.vi"("error in (no error)"=w524, "Channel in"=w523) -> ("error out"=w520:errorcluster, "GUI request"=w522:T2)  [unwired: 7 in, 1 out]
          n220 = Unbundle By Name(w522) -> ("field 2"=w521:string, "field 3"=w519:string)
          n221 = case shown="\"WAVEPLATE_POS\"" w521 {
            tunnel: [w539 w546 w562 w581 w595 w606] -> w528
            tunnel: w523 -> [w539 w541 w569 w586 w599 w608]
            tunnel: [w538 w545 w561 w580 w593 w605] -> w525
            tunnel: w520 -> [w538 w550 w570 w585 w594 w600]
            tunnel: w519 -> [_ w551 w571 w591 w597 w609]
            frame "False", Default {
            }
            frame "EXPTIME" {
              n222 = call-dynamic "Read Classes.vi"("error in (no error)"=w550, "Channel in"=w541) -> ("error out"=w549:errorcluster, "Classes"=w544:T1, "Channel out"=w540:refnum<class "SPARC4_Channel.lvclass">)  [unwired: 7 in]
              n223 = Unbundle By Name(w544) -> ("Sim_CCD.lvclass"=w548:refnum<class "Sim_CCD.lvclass">)
              n224 = Fract/Exp String To Number(string=w551, default (0 dbl)=0.0) -> (number=w558:dbl)  [unwired: 2 in, 1 out]
              n225 = call "read new acquisition config.vi"("error in (no error)"=w549, "Simulated_CCD_Camera in"=w548) -> ("error out"=w554:errorcluster, "New SET parameters"=w557:cluster{"EXPTIME":dbl, "#FRAMES":u32}, "Simulated_CCD_Camera out"=w555:refnum<class "Sim_CCD.lvclass">)  [unwired: 7 in]
              n226 = Bundle By Name(cluster=w557, "EXPTIME"=w558) -> (w556:cluster{"EXPTIME":dbl, "#FRAMES":u32})
              n227 = call "write new acquisition config.vi"("error in (no error)"=w554, "new acquisition configuration"=w556, "Simulated_CCD_Camera in"=w555) -> ("error out"=w553:errorcluster, "Simulated_CCD_Camera out"=w552:refnum<class "Sim_CCD.lvclass">)  [unwired: 7 in]
              n228 = call-dynamic "verify expouse time.vi"("error in (no error)"=w553, "Simulated_CCD_Camera in"=w552) -> ("error out"=w547:errorcluster, "Simulated_CCD_Camera out"=w542:refnum<class "Sim_CCD.lvclass">)  [unwired: 8 in]
              n229 = Bundle By Name(cluster=w544, "Sim_CCD.lvclass"=w542) -> (w543:T1)
              n230 = call-dynamic "Write Classes.vi"("error in (no error)"=w547, "Classes"=w543, "Channel in"=w540) -> ("error out"=w545:errorcluster, "Channel out"=w546:refnum<class "SPARC4_Channel.lvclass">)  [unwired: 7 in]
            }
            frame "#FRAMES" {
              n231 = call-dynamic "Read Classes.vi"("error in (no error)"=w570, "Channel in"=w569) -> ("error out"=w567:errorcluster, "Classes"=w565:T1, "Channel out"=w560:refnum<class "SPARC4_Channel.lvclass">)  [unwired: 7 in]
              n232 = Unbundle By Name(w565) -> ("Sim_CCD.lvclass"=w568:refnum<class "Sim_CCD.lvclass">)
              n233 = Fract/Exp String To Number(string=w571, default (0 dbl)=u32 0) -> (number=w572:u32)  [unwired: 2 in, 1 out]
              n234 = call "read new acquisition config.vi"("error in (no error)"=w567, "Simulated_CCD_Camera in"=w568) -> ("error out"=w575:errorcluster, "New SET parameters"=w578:cluster{"EXPTIME":dbl, "#FRAMES":u32}, "Simulated_CCD_Camera out"=w576:refnum<class "Sim_CCD.lvclass">)  [unwired: 7 in]
              n235 = Bundle By Name(cluster=w578, "#FRAMES"=w572) -> (w577:cluster{"EXPTIME":dbl, "#FRAMES":u32})
              n236 = call "write new acquisition config.vi"("error in (no error)"=w575, "new acquisition configuration"=w577, "Simulated_CCD_Camera in"=w576) -> ("error out"=w573:errorcluster, "Simulated_CCD_Camera out"=w574:refnum<class "Sim_CCD.lvclass">)  [unwired: 7 in]
              n237 = call "verify #frames.vi"("error in (no error)"=w573, "Simulated_CCD_Camera in"=w574) -> ("error out"=w566:errorcluster, "Simulated_CCD_Camera out"=w564:refnum<class "Sim_CCD.lvclass">)  [unwired: 8 in]
              n238 = Bundle By Name(cluster=w565, "Sim_CCD.lvclass"=w564) -> (w563:T1)
              n239 = call-dynamic "Write Classes.vi"("error in (no error)"=w566, "Classes"=w563, "Channel in"=w560) -> ("error out"=w561:errorcluster, "Channel out"=w562:refnum<class "SPARC4_Channel.lvclass">)  [unwired: 7 in]
            }
            frame "#CYCLES" {
              n240 = Fract/Exp String To Number(string=w591, default (0 dbl)=u32 0) -> (number=w589:u32)  [unwired: 2 in, 1 out]
              n241 = call-dynamic "read new acq config.vi"("error in (no error)"=w585, "Channel in"=w586) -> ("error out"=w588:errorcluster, "new acq config"=w590:cluster{"suffix":string, "#CYCLES":u32}, "Channel out"=w587:refnum<class "SPARC4_Channel.lvclass">)  [unwired: 7 in]
              n242 = Bundle By Name(cluster=w590, "#CYCLES"=w589) -> (w584:cluster{"suffix":string, "#CYCLES":u32})
              n243 = call-dynamic "Write new acq config.vi"("error in (no error)"=w588, "new acq config"=w584, "Channel in"=w587) -> ("error out"=w583:errorcluster, "Channel out"=w582:refnum<class "SPARC4_Channel.lvclass">)  [unwired: 7 in]
              n244 = call "verify #cycles.vi"("error in (no error)"=w583, "Channel in"=w582) -> ("error out"=w580:errorcluster, "Channel out"=w581:refnum<class "SPARC4_Channel.lvclass">)  [unwired: 8 in]
            }
            frame "WAVEPLATE_POS" {
              n245 = Decimal String To Number(string=w597) -> (number=w598:i32)  [unwired: 2 in, 1 out]
              n246 = Bundle By Name(cluster=w599, "WAVEPLATE_POS"=w598) -> (w596:refnum<class "SPARC4_Channel.lvclass">)
              n247 = call "verify waveplate_pos.vi"("error in (no error)"=w594, "SPARC4_Channel in"=w596) -> ("error out"=w593:errorcluster, "SPARC4_Channel out"=w595:refnum<class "SPARC4_Channel.lvclass">)  [unwired: 8 in]
            }
            frame "SUFFIX" {
              n248 = To Lower Case(string=w609) -> (all lower case string=w602:string)
              n249 = call-dynamic "read new acq config.vi"("error in (no error)"=w600, "Channel in"=w608) -> ("error out"=w604:errorcluster, "new acq config"=w603:cluster{"suffix":string, "#CYCLES":u32}, "Channel out"=w607:refnum<class "SPARC4_Channel.lvclass">)  [unwired: 7 in]
              n250 = Bundle By Name(cluster=w603, "suffix"=w602) -> (w601:cluster{"suffix":string, "#CYCLES":u32})
              n251 = call-dynamic "Write new acq config.vi"("error in (no error)"=w604, "new acq config"=w601, "Channel in"=w607) -> ("error out"=w605:errorcluster, "Channel out"=w606:refnum<class "SPARC4_Channel.lvclass">)  [unwired: 7 in]
            }
          }
          n252 = call-dynamic "update camera op mode error.vi"("error in (no error)"=w525, "SPARC4_Channel in"=w528) -> ("error out"=w529:errorcluster, "SPARC4_Channel out"=w530:refnum<class "SPARC4_Channel.lvclass">)  [unwired: 8 in]
          n253 = call-dynamic "log acq config errors.vi"("error in (no error)"=w529, "SPARC4_Channel in"=w530) -> ("error out"=w526:errorcluster, "SPARC4_Channel out"=w527:refnum<class "SPARC4_Channel.lvclass">)  [unwired: 8 in]
          n254 = call "write acquisition config.vi"("error in (no error)"=w526, "Channel in"=w527) -> ("error out"=w532:errorcluster, "Channel out"=w531:refnum<class "SPARC4_Channel.lvclass">)  [unwired: 8 in]
          n255 = call-dynamic "Send status.vi"("error in (no error)"=w532, "Channel in"=w531) -> ("error out"=w536:errorcluster, "Channel out"=w537:refnum<class "SPARC4_Channel.lvclass">)  [unwired: 8 in]
          n256 = call "write state.vi"("error in (no error)"=w536, "state"="False", "Channel in"=w537) -> ("error out"=w534:errorcluster, "Channel out"=w535:refnum<class "SPARC4_Channel.lvclass">)  [unwired: 7 in]
        }
      }
    }
    frame Error {
    }
  }
  "error out" <- w3
  "Channel out" <- w1
